vi "Encode Parameter and Update Word (32-bit).vi"(8 "error in":errorcluster, 9 "parameter definition":T1={"start index"=10, "size"=19, "encoding"=enum."BNR", "signed"=FALSE, "scale multiplier"=1.0, "scale offset"=0.0, "default value"=0.0}, 10 "parameter value":dbl, 11 "word in":u32 format="%032b") -> (0 "error out":errorcluster, 3 "word out":u32 format="%032b")   [LabVIEW 2020]
uses:
  Parameter Definition.ctl
  <vilib>/NI/NI VeriStand Encoding and Decoding/Encoding.ctl
  <vilib>/NI/NI VeriStand Encoding and Decoding/Parity.ctl
  1445f95d-237d-4fc6-96b9-8992d347f513.vi
  6b8853f0-8e5d-49e3-9391-4d3f8e5314b0.vi
  2babc4f4-546e-4d35-846d-a4a1fbac0249.vi
  1445f95d-237d-4fc6-96b9-8992d347f513.vi/9377bb8f-44b5-4a8f-87f1-966fd5a9edcc.vi
  1445f95d-237d-4fc6-96b9-8992d347f513.vi/e95d9d1f-307c-44d6-9f26-c3f519a4990d.vi
  1445f95d-237d-4fc6-96b9-8992d347f513.vi/0c23f515-4369-4514-bc3d-4444e6b437b2.vi
  6b8853f0-8e5d-49e3-9391-4d3f8e5314b0.vi/136dcdcb-2dd3-4a4d-a796-a8f7a3f8e1ac.vi
  6b8853f0-8e5d-49e3-9391-4d3f8e5314b0.vi/a54b505c-1216-4ef4-8378-3ceda9d188df.vi
  <vilib>/NI/NI VeriStand Encoding and Decoding/Get Bits Per Digit from Base.vi
  <vilib>/NI/NI VeriStand Encoding and Decoding/Encoding and Decoding.lvlib
panel:
  # "P (1) | SSM (2) | Parameter (19) | SDI (2) | LABEL (8)"
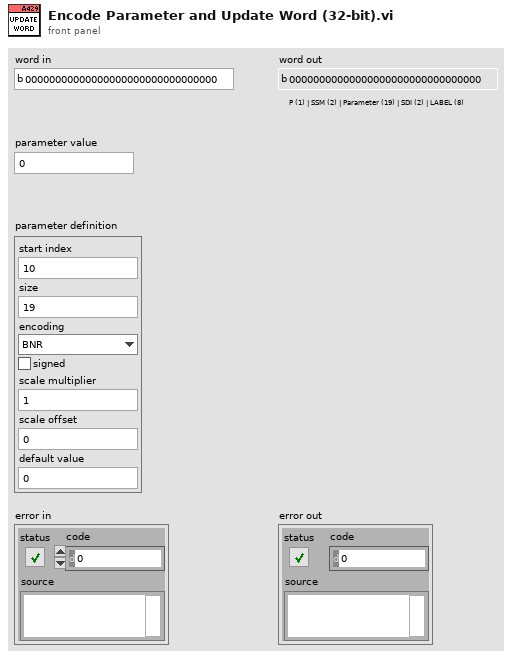
[diagram p1: front panel]
types:
  T1 = typedef "Parameter Definition.ctl" = cluster{"start index":i32, "size":i32, "encoding":T2, "signed":bool, "scale multiplier":dbl, "scale offset":dbl, "default value":dbl}
  T2 = typedef "Encoding and Decoding.lvlib/Encoding.ctl" = enum16{"BNR", "BCD", "Discrete"}
  T3 = typedef "Encoding and Decoding.lvlib/Parity.ctl" = enum16{"Even", "Odd"}
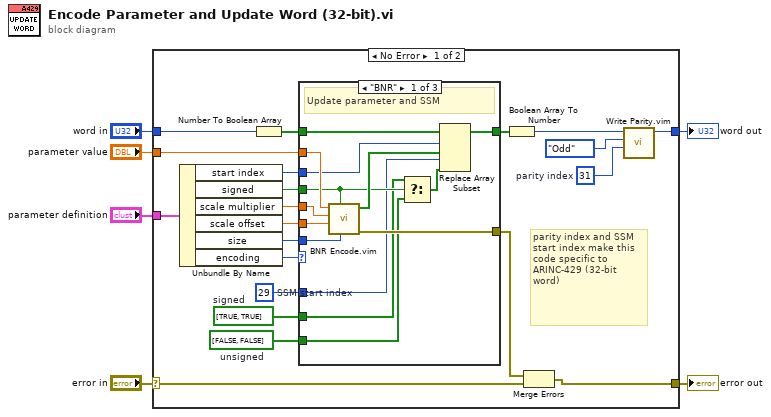
[diagram p0: block diagram]
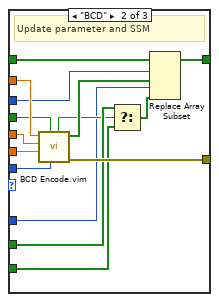
[diagram p2: hidden frame]
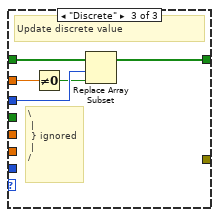
[diagram p3: hidden frame]
diagram:
  n1 = case shown="No Error" "error in" {
    selector: "error in" -> [w13 w62]
    tunnel: "parameter value" -> [w20 _]
    tunnel: "word in" -> [w19 w63]
    tunnel: "parameter definition" -> [w18 _]
    tunnel: [w8 w63] -> w3
    tunnel: [w12 w62] -> w1
    frame No Error {
      w7 = 31  # parity index
      w15 = 29  # SSM start index
      w17 = bool[] [TRUE, TRUE]  # signed
      w16 = bool[] [FALSE, FALSE]  # unsigned
      # "parity index and SSM start index make this code specific to ARINC-429 (32-bit word)"
      n2 = Unbundle By Name(w18) -> ("start index"=w21:i32, "signed"=w22:bool, "scale multiplier"=w25:dbl, "scale offset"=w24:dbl, "size"=w23:i32, "encoding"=w27:T2)
      n3 = Number To Boolean Array(number=w19) -> (Boolean array=w26:bool[])
      n4 = case shown="\"BNR\"" w27 {
        tunnel: w20 -> [w41 w56 w61]
        tunnel: w25 -> [w40 w55 _]
        tunnel: w24 -> [w39 w54 _]
        tunnel: w23 -> [w38 w52 _]
        tunnel: w22 -> [w32 w53 _]
        tunnel: [w37 w51 _] -> w14
        tunnel: w21 -> [w35 w49 w60]
        tunnel: w26 -> [w34 w50 w58]
        tunnel: [w33 w42 w57] -> w10
        tunnel: w17 -> [w31 w47 _]
        tunnel: w16 -> [w30 w46 _]
        tunnel: w15 -> [w29 w43 _]
        frame "BNR" {
          # "Update parameter and SSM"
          n5 = call "BNR Encode.vim"("data size (bits)"=w38, "signed"=w32, "scale offset"=w39, "scale multiplier"=w40, "value"=w41) -> ("error out"=w37:errorcluster, "BNR encoded value"=w36:bool[])  [unwired: 5 in]
          n6 = Select(t=w31, s=w32, f=w30) -> (s? t:f=w28:bool[])
          n7 = Replace Array Subset(array=w34, new element #1=w36, index #1=w35, new element #2=w28, index #2=w29) -> (w33:bool[])
        }
        frame "BCD" {
          # "Update parameter and SSM"
          n8 = call "BCD Encode.vim"("data size (bits)"=w52, "signed"=w53, "scale offset"=w54, "scale multiplier"=w55, "value"=w56) -> ("error out"=w51:errorcluster, "BCD encoded value"=w48:bool[], "signed?"=w45:bool)  [unwired: 4 in]
          n9 = Select(t=w47, s=w45, f=w46) -> (s? t:f=w44:bool[])
          n10 = Replace Array Subset(array=w50, new element #1=w48, index #1=w49, new element #2=w44, index #2=w43) -> (w42:bool[])
        }
        frame "Discrete" {
          # "\\\n |\n } ignored \n |\n/"
          # "Update discrete value"
          n11 = Not Equal To 0?(x=w61) -> (x != 0?=w59:bool)
          n12 = Replace Array Subset(array=w58, new element=w59, index=w60) -> (w57:bool[])
        }
      }
      n13 = Boolean Array To Number(Boolean array=w10) -> (number=w9:u32)
      n14 = Merge Errors(w14, w13) -> (w12:errorcluster)
      n15 = call "Write Parity.vim"("parity index"=w7, "parity"=Parity."Odd", "word in"=w9) -> ("word out"=w8:u32)  [unwired: 8 in]
    }
    frame Error {
    }
  }
  "word out" <- w3
  "error out" <- w1
